vi "Toggle.vi"(1 "Input":bool) -> (0 "Output":bool)   [LabVIEW 2017]
panel:
  out "Toggle5":bool
  out "Toggle4":bool
  out "Toggle3":bool
  out "Toggle2":bool
  out "Toggle":bool
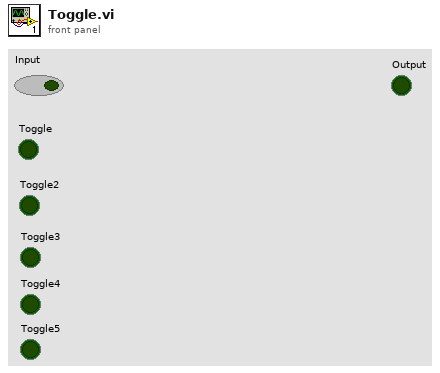
[diagram p1: front panel]
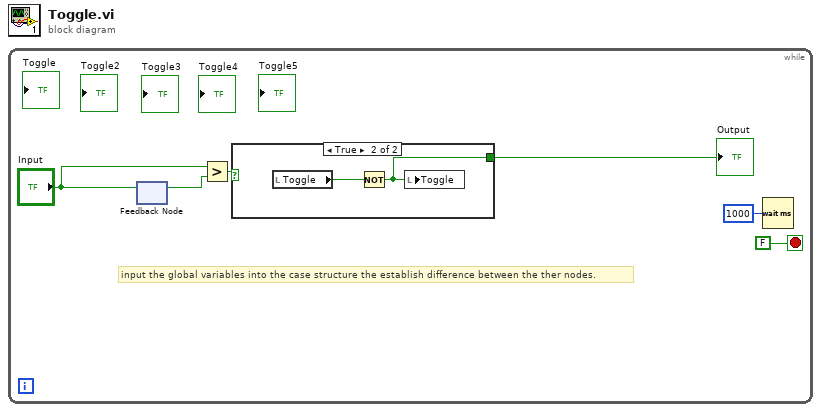
[diagram p0: block diagram]
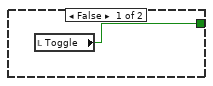
[diagram p2: hidden frame]
diagram:
  n1 = while {
    stop <- FALSE stop-if-true
    # "input the global variables into the case structure the establish difference between the ther nodes."
    n2 = feedback-in #1("Input") -> ()
    n3 = feedback #1() -> (w4:bool)  [unwired: 1 in]
    n4 = Greater?(x="Input", y=w4) -> (0:w3:bool)
    n5 = case shown="True" w3 {
      tunnel: [w7 w9] -> w2
      frame False {
        n6 = local read "Toggle"() -> (w7:bool)
      }
      frame True {
        n7 = local read "Toggle"() -> (w8:bool)
        n8 = Not(x=w8) -> (.not. x?=w9:bool)
        n9 = local write "Toggle"(w9) -> ()
      }
    }
    "Output" <- w2
    n10 = Wait (ms)(milliseconds to wait=u32 1000) -> ()  [unwired: 1 out]
  }
